vi "swin.vi"(8 "error in (no error)":errorcluster, 11 "ModelDuck in":refnum<class "ModelDuck.lvclass">) -> (0 "error out":errorcluster, 2 "State":string, 3 "ModelDuck out":refnum<class "ModelDuck.lvclass">)   [LabVIEW 2013, in "ModelDuck.lvclass"]
uses:
  ModelDuck.lvclass
  Duck/Duck.lvclass
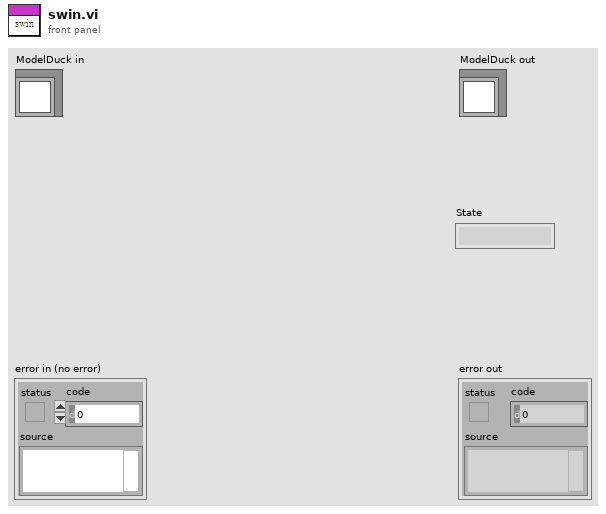
[diagram p1: front panel]
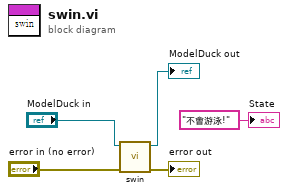
[diagram p0: block diagram]
diagram:
  n1 = call-parent "swin.vi"("error in (no error)"="error in (no error)", "Duck in"="ModelDuck in") -> ("error out"=→"error out":errorcluster, "Duck out"=→"ModelDuck out":refnum<class "ModelDuck.lvclass">)  [unwired: 7 in, 1 out]
  "State" <- "不會游泳!" ("State")
